vi "HighlightByUID.vi"(0 "__args":cluster{"targetVi":string, "UID":i32}) -> (1 "__return":cluster{"UID":i32, "UID":i32}, 2 "__errStatus":bool, 3 "__errCode":i32, 4 "__errSource":string)   [LabVIEW 2013]
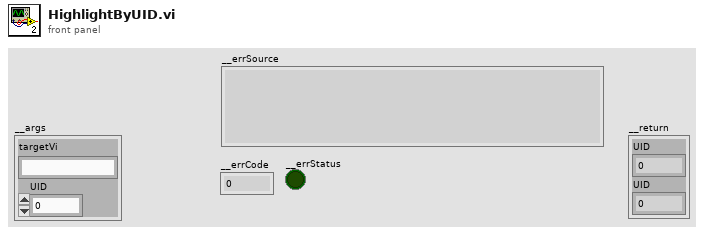
[diagram p1: front panel]
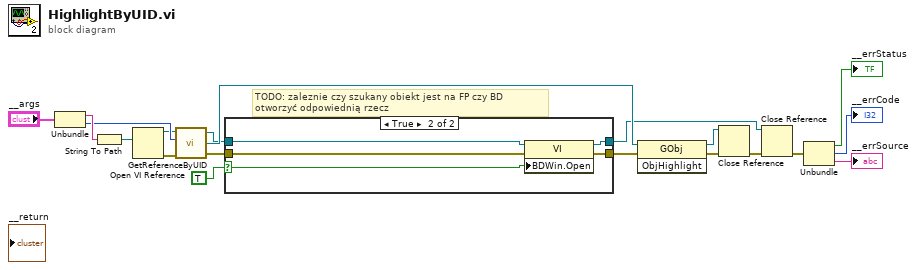
[diagram p0: block diagram]
diagram:
  # "TODO: zaleznie czy szukany obiekt jest na FP czy BD\notworzyć odpowiednią rzecz"
  n1 = Unbundle("__args") -> ("targetVi"=w14:string, "UID"=w10:i32)
  n2 = String To Path(string=w14) -> (path=w15:path)
  n3 = Open VI Reference(vi path=w15) -> (vi reference=w7:refnum<vi>, error out=w3:errorcluster)  [unwired: 5 in]
  n4 = call "GetReferenceByUID.vi"("error in (no error)"=w3, "UID"=w10, "targetVI"=w7) -> ("error out"=w4:errorcluster, "refNum"=w12:refnum<vi>, "dup targetVI"=w6:refnum<vi>)  [unwired: 1 in]
  n5 = case shown="True" TRUE ("Block Diagram Window:Open") {
    selector: TRUE ("Block Diagram Window:Open") -> [_ w22]
    tunnel: w6 -> [w21 w26]
    tunnel: [w20 w25] -> w5
    tunnel: w4 -> [w20 w24]
    tunnel: [w21 w23] -> w2
    frame False {
    }
    frame True {
      n6 = property class="VI"(reference=w26, error in=w24, "BDWin.Open"=w22) -> (reference out=w23:refnum<vi>, error out=w25:errorcluster)
    }
  }
  n7 = invoke class="GObj" method="ObjHighlight"(reference=w12, error in=w5) -> (reference out=w11:refnum<vi>, error out=w9:errorcluster)  [unwired: 1 in, 1 out]
  n8 = Close Reference(reference=w11, error in (no error)=w9) -> (error out=w8:errorcluster)
  n9 = Close Reference(reference=w2, error in (no error)=w8) -> (error out=w13:errorcluster)
  n10 = Unbundle(w13) -> ("status"=→"__errStatus":bool, "code"=→"__errCode":i32, "source"=→"__errSource":string)
